vi "Help UI.vi"   [LabVIEW 2020, in "App.lvlib" / "MazeUI.lvclass"]
uses:
  MazeUI.lvclass
panel:
  # "1. The Maze App will initially open with a demo mouse implementation that performs wall following.\n\n2. Mouse Name is the project name you enter when you create a new Maze project.\n\n3. Make sure you set your name in the Author property within the Mouse instance you create.\n\n4. Click load mouse to browse to your built LLB to test your mouse implementation. See below for information on starting a new project.\n\n5. If you implemented a configuration UI, you can open it to change how your mouse makes its decisions. When loading different mouse implementations or opening the Maze App again the mouse will be back at its default config. When submitting the mouse for scoring we will only be using your mouse with whatever its defaults are saved as.\n\n6. Random Maze will generate a new maze for you to test with. If you want to keep a maze that you can re-use later, you can use the save and load buttons to save mazes to disk to be reloaded again later."
  # "You are here!"
  # "Status shows you whether the maze hasn't been started (Idle), is currently in progress (Running), was successful and reached the goal, or attempted to make an invalid action."
  # "Run and Stop control the running state of the maze. Run starts the maze and lets it keep running until it completes or has an issue. Anytime Stop is clicked the maze will be reset and the mouse will start over at the beginning for the current maze."
  # "Actions shows you the number of times the Decide Action VI in a mouse was called. The actions are turning, moving forward a step, placing a marker, and picking up a marker."
  # "Step performs a single action decision for a mouse. This can be useful to closely watch its behavior. Step can be pressed while in run mode to pause the run and single-step but to start running again the maze needs to be reset."
  # "Reset sets the current maze back to its beginning state."
  # "Move the Run Speed slider to change how quickly the maze is run when the Run button is pressed. Moving the slider all the way to the right runs the maze as fast as the computer can manage."
  # "To start a new maze solver project, start by opening the Create Project dialog. This can be done by clicking the Create Project button on LabVIEW's Getting Started Window or selecting Create Project from the File menu in any LabVIEW window."
  # "There is a Summer of LabVIEW - Maze project template that you can start with to ensure you're setup with the proper inheritance and build spec. There will be a readme in the project for futher steps."
  # "Creating a new solver project:"
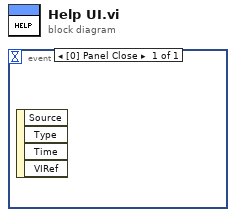
[diagram p0: block diagram]
diagram:
  n1 = event shown="[0] Panel Close" {
    selector: _ -> [_]
    dyn-events: _ -> [_]
    timeout: _ -> [_]
    event Panel Close {
      n2 = event-data() -> ()  [unwired: 1 in, 4 out]
    }
  }
